vi "Test_Hysteresis_min-LAPTOP-A1ILEVN9.vi"() -> ()   [LabVIEW 2022 SP3]
panel:
  in  "type":enum16{"percentage", "level"}(ring)
  out "Deviation":bool
  in  "H":dbl=22.0 format="%#_13g"
  in  "Min":dbl=26.0 format="%#_13g"
  in  "input":dbl
  in  "stop":bool
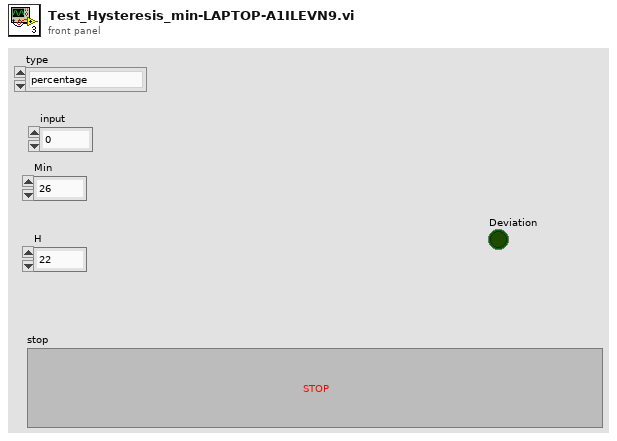
[diagram p1: front panel]
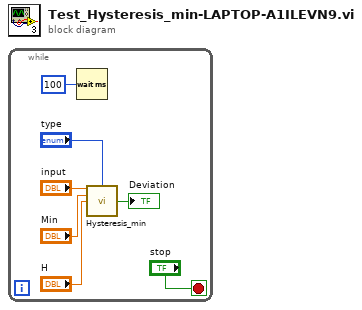
[diagram p0: block diagram]
diagram:
  n1 = while {
    stop <- "stop" stop-if-true
    n2 = Wait (ms)(milliseconds to wait=u32 100) -> ()  [unwired: 1 out]
    n3 = call "Hysteresis_min.vi"("input"="input", "type"="type", "Min"="Min", "H"="H") -> ("Deviation"=→"Deviation":bool)  [unwired: 10 in, 1 out]
  }
